vi "get id hash string.vi"(8 "error in (no error)":errorcluster, 11 "id":variant) -> (0 "error out":errorcluster, 3 "String":string)   [LabVIEW 2017, in "JSONRPC Server.lvclass"]
uses:
  JSONRPC Server.lvclass
  <vilib>/National Instruments/Variant JSON API/Variant JSON API.lvlib
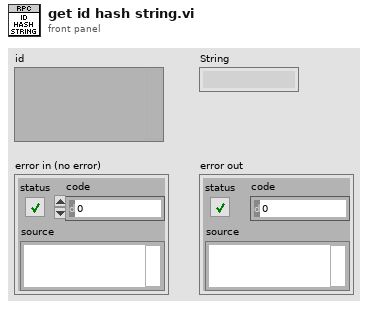
[diagram p1: front panel]
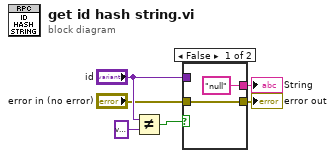
[diagram p0: block diagram]
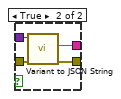
[diagram p2: hidden frame]
diagram:
  n1 = Not Equal?(x="id", y=variant) -> (x != y?=w6:bool)
  n2 = case shown="False" w6 {
    tunnel: ["null" ("String") w12] -> w1
    tunnel: [w7 w11] -> w2
    tunnel: "error in (no error)" -> [w7 w10]
    tunnel: "id" -> [_ w9]
    frame False {
    }
    frame True {
      n3 = call <vilib>:"Variant to JSON String.vi"("error in (no error)"=w10, "Variant in"=w9) -> ("error out"=w11:errorcluster, "String"=w12:string)  [unwired: 7 in, 1 out]
    }
  }
  "error out" <- w2
  "String" <- w1
